vi "Write Actual Transition Time.vi"(8 "error in (no error)":errorcluster, 10 "actual transition time":dbl, 11 "signal configuration in":refnum<class "SV Signal.lvclass">) -> (0 "error out":errorcluster, 3 "signal configuration out":refnum<class "SV Signal.lvclass">)   [LabVIEW 2017, in "SV Signal.lvclass"]
uses:
  <vilib>/addons/_NISVFA/_Generation/Signal Generation/SV Signal/SV Signal.lvclass
  <vilib>/addons/_NISVFA/_Generation/Signal Generation/SV Signal/sv_Signal State Attribute.ctl
  <vilib>/addons/_NISVFA/_Generation/Signal Generation/SV Signal/SV Signal.lvclass/SV Signal.ctl
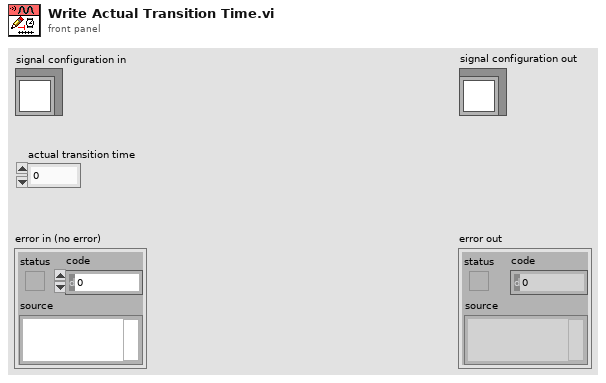
[diagram p1: front panel]
types:
  T1 = typedef "SV Signal.lvclass/sv_Signal State Attribute.ctl" = string
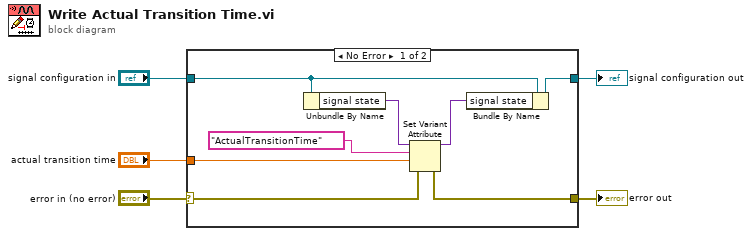
[diagram p0: block diagram]
diagram:
  n1 = case shown="No Error" "error in (no error)" {
    selector: "error in (no error)" -> [w9 w15]
    tunnel: [w8 w15] -> w4
    tunnel: [w10 w14] -> w2
    tunnel: "signal configuration in" -> [w11 w14]
    tunnel: "actual transition time" -> [w7 _]
    frame No Error {
      n2 = Unbundle By Name(w11) -> ("signal state"=w12:variant)
      n3 = Set Variant Attribute(Variant=w12, name=T1 "ActualTransitionTime" ("attribute"), value=w7, error in=w9) -> (Variant out=w13:variant, error out=w8:errorcluster)  [unwired: 1 out]
      n4 = Bundle By Name(cluster=w11, "signal state"=w13) -> (w10:refnum<class "SV Signal.lvclass">)
    }
    frame Error {
    }
  }
  "error out" <- w4
  "signal configuration out" <- w2
